vi "State Logic.vi"(0 "TLB' data in":refnum<class "{TMPL} TLB`.lvclass">, 1 "process state logic enable":bool, 5 "trigger queue in":refnum<queue>, 7 "action queue in":refnum<queue>, 11 "error in":errorcluster) -> (4 "TLB' data out":refnum<class "{TMPL} TLB`.lvclass">, 15 "error out":errorcluster)   [LabVIEW 2023, in "TLB` InstStu GPlugin Template.lvlib" / "{TMPL} TLB`.lvclass"]
doc: "Control process for TLB' template.\n\n<B>Input Parameters</B>\n\n<B>TLB' data in</B> is the templates' private data.\n\n<B>process state logic enable</B> enable state logic change.\n\n<B>trigger queue in</B> is a reference to a queue. Use the Create Trigger Queue function to obtain a queue reference. \n\n<B>action queue in</B> is a reference to a queue. Use the Create Action Queue function to obtain a queue reference. \n\n<B>timeout (ms)</B> queue timeout.\n\n<B>error in</B> describes error conditions that occur before this node runs. This input provides standard error in functionality.\n\n<B>Output Parameters</B>\n\n<B>TLB' data out</B> is the templates' private data.\n\n<B>error out</B> contains error information. This output provides standard error out functionality."
uses:
  {TMPL} TLB`.lvclass
  Application Components/Trigger API/System Trigger Element.ctl
  Application Components/Trigger API/System Trigger.ctl
  Core Components/Actions/System Action Element.ctl
  {TMPL} TLB`.lvclass/{TMPL} TLB`.ctl
  State.ctl
  Core Components/Error Handler/TLB` Error Handler.lvclass/TLB` Error Handler.ctl
  Core Components/Error Handler/accessors/Get Action Causing Error.vi
  Core Components/Error Handler/accessors/Get Originating State.vi
  Core Components/Error Handler/accessors/Get Destination State.vi
  Core Components/Error Handler/accessors/Get Executed System Actions.vi
  Core Components/Error Handler/accessors/Get Remaing System Actions.vi
  Core Components/Error Handler/Core/actions/support/Error FLUSH-LOG-DIALOG.vi
  Core Components/Error Handler/Core/actions/support/Error FLUSH-DIALOG.vi
  Application Components/Trigger API/{TMPL} Trigger API.lvlib
  Core Components/Error Handler/TLB` Error Handler.lvclass
  Core Components/Actions/Actions.lvlib
  TLB` InstStu GPlugin Template.lvlib
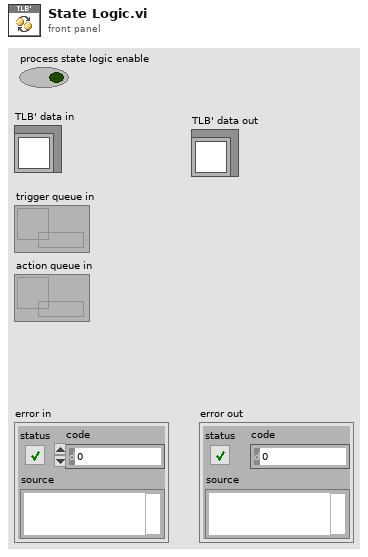
[diagram p1: front panel]
types:
  T1 = typedef "TLB` InstStu GPlugin Template.lvlib/{TMPL} TLB`.lvclass/State.ctl" = enum16{"<Startup>", "Idle", "Connected", "Monitoring", "<Shutdown>", "<Error>"}
  T2 = typedef "TLB` InstStu GPlugin Template.lvlib/{TMPL} Trigger API.lvlib/System Trigger.ctl" = enum16{"<None>", "Connect", "Start Acquisition", "Stop Acquisition", "Disconnect", "Load Configuration", "Save Configuration", "<Return to Safe State Actions>", "<Cache User Parameters>", "<Close Application>", "<Error>"}
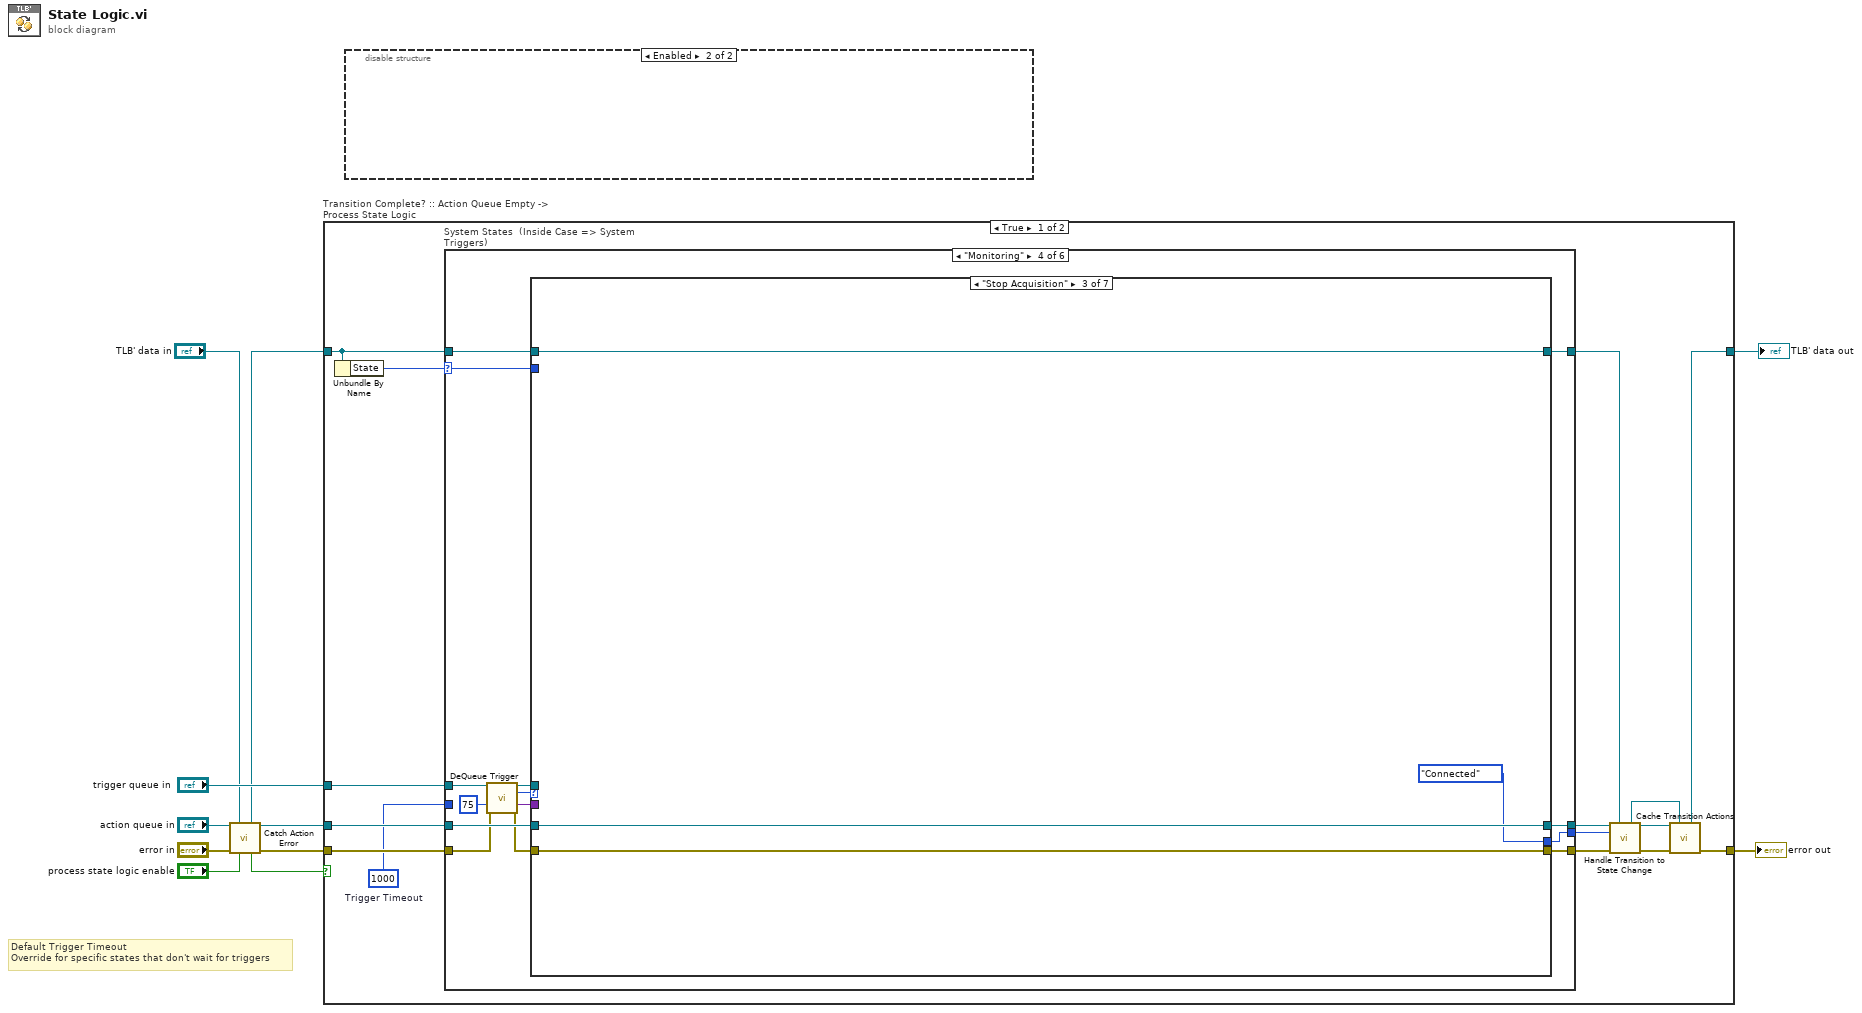
[diagram p0: block diagram]
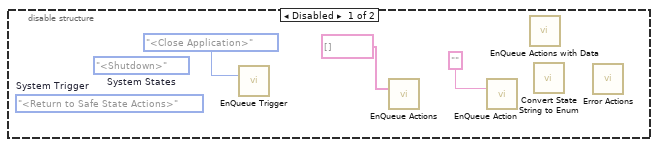
[diagram p2: hidden frame]
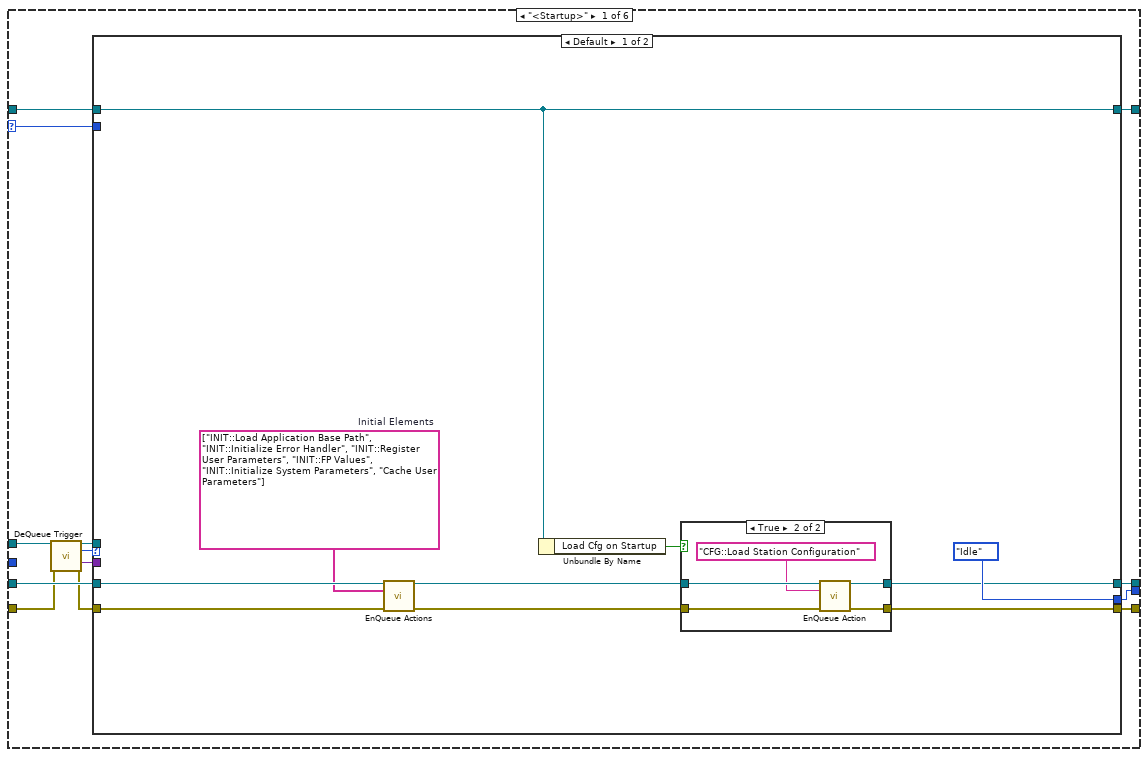
[diagram p3: hidden frame]
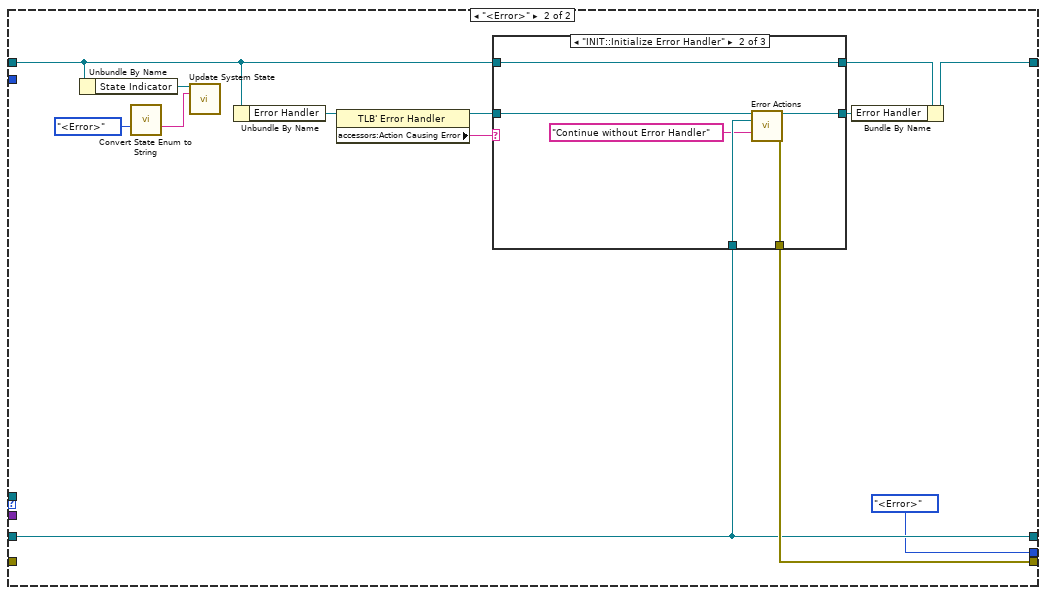
[diagram p5: hidden frame]
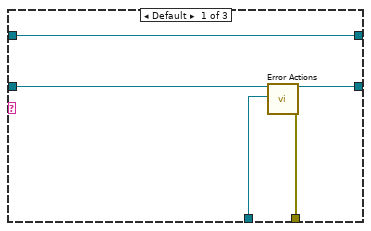
[diagram p6: hidden frame]
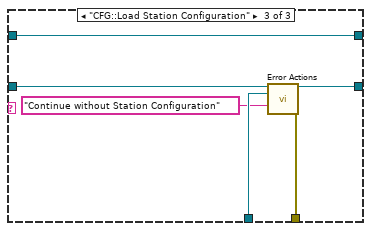
[diagram p7: hidden frame]
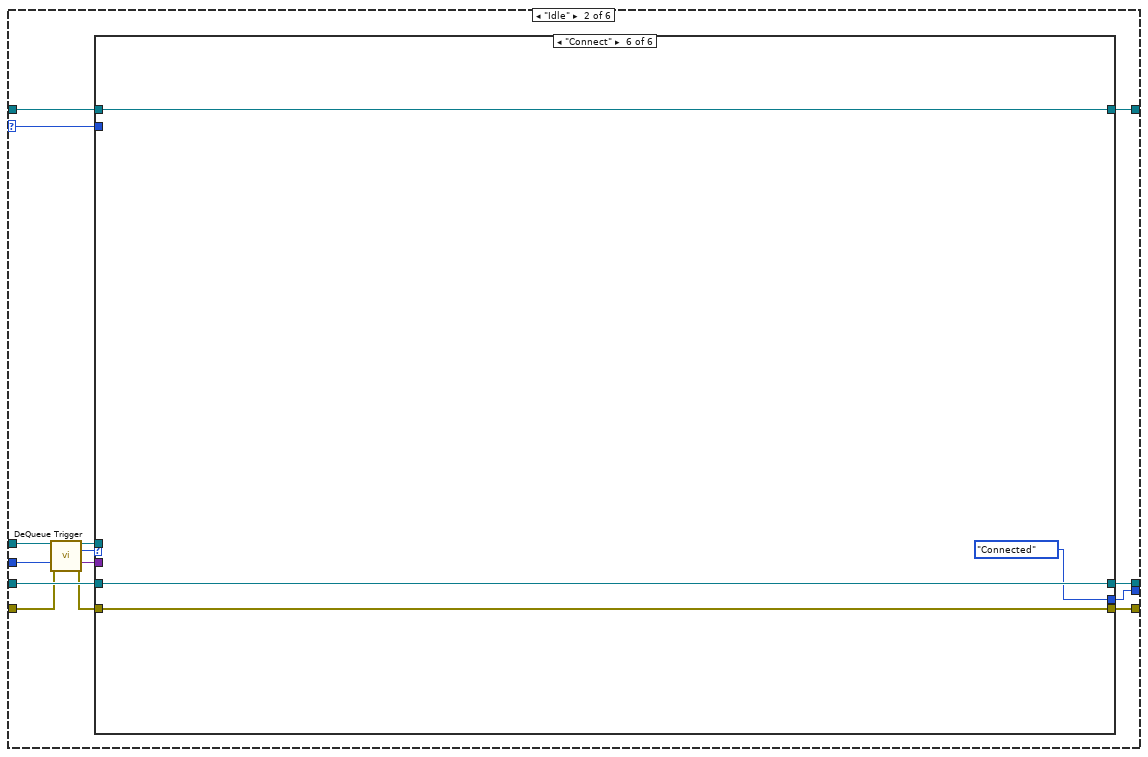
[diagram p8: hidden frame]
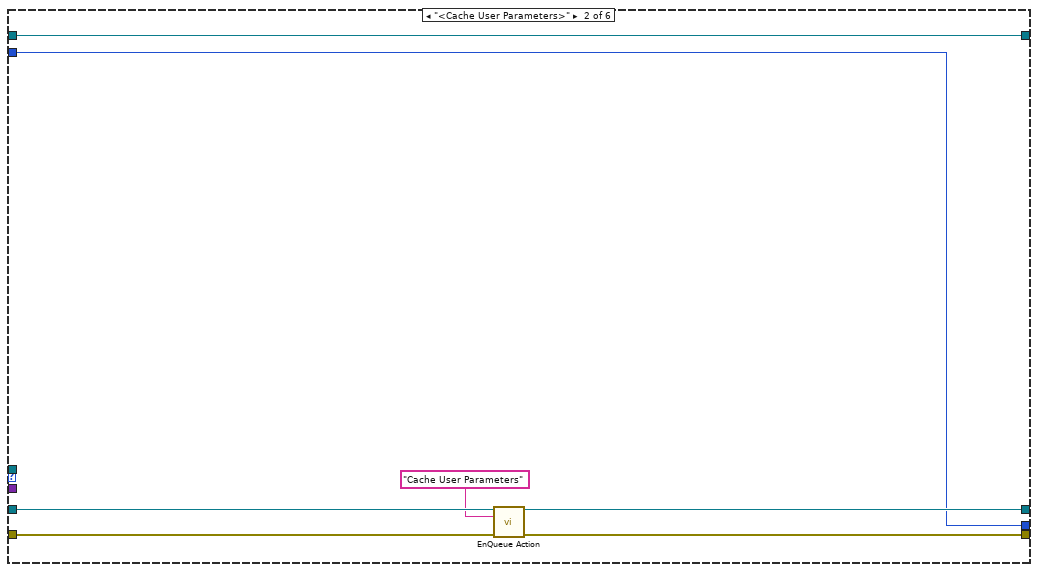
[diagram p10: hidden frame]
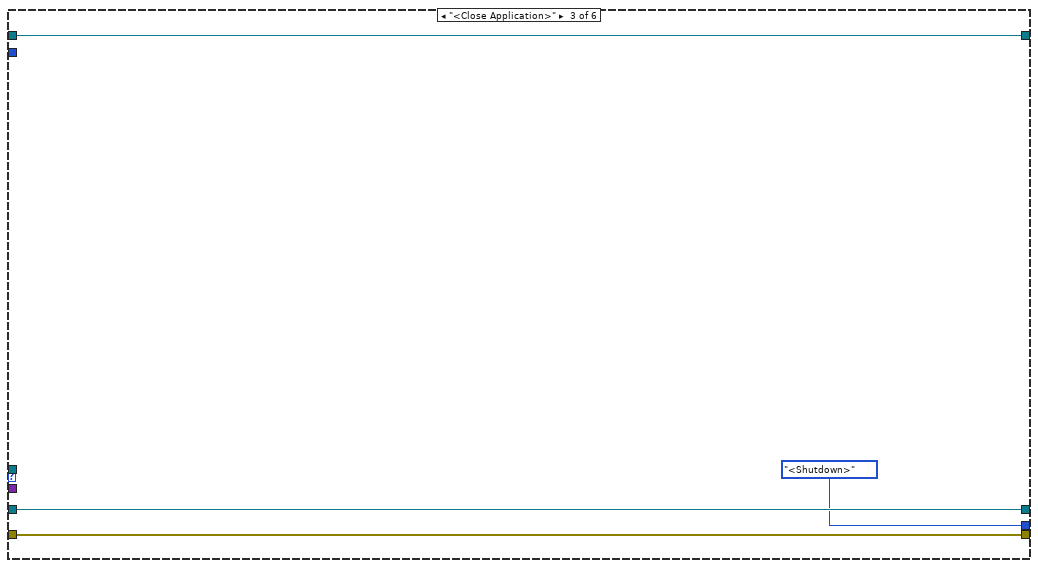
[diagram p11: hidden frame]
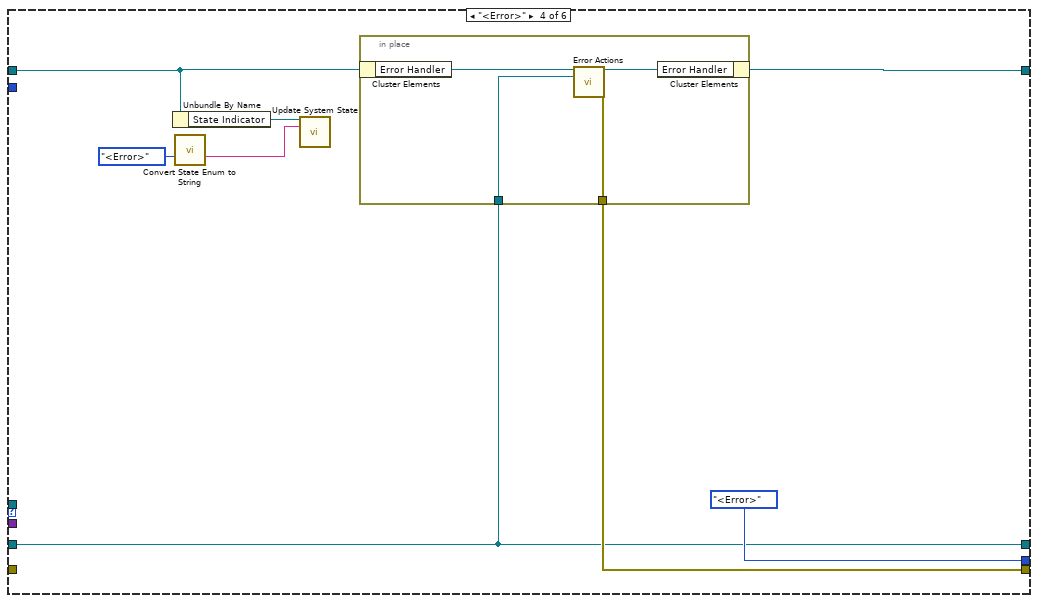
[diagram p12: hidden frame]
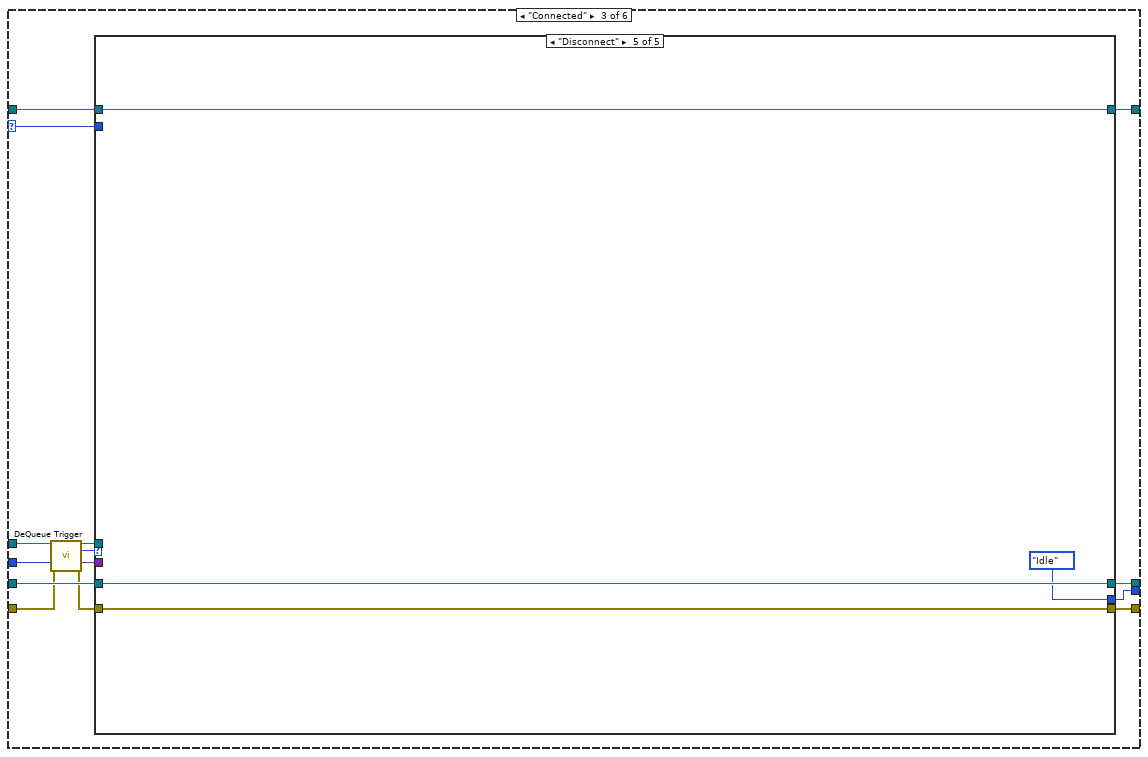
[diagram p14: hidden frame]
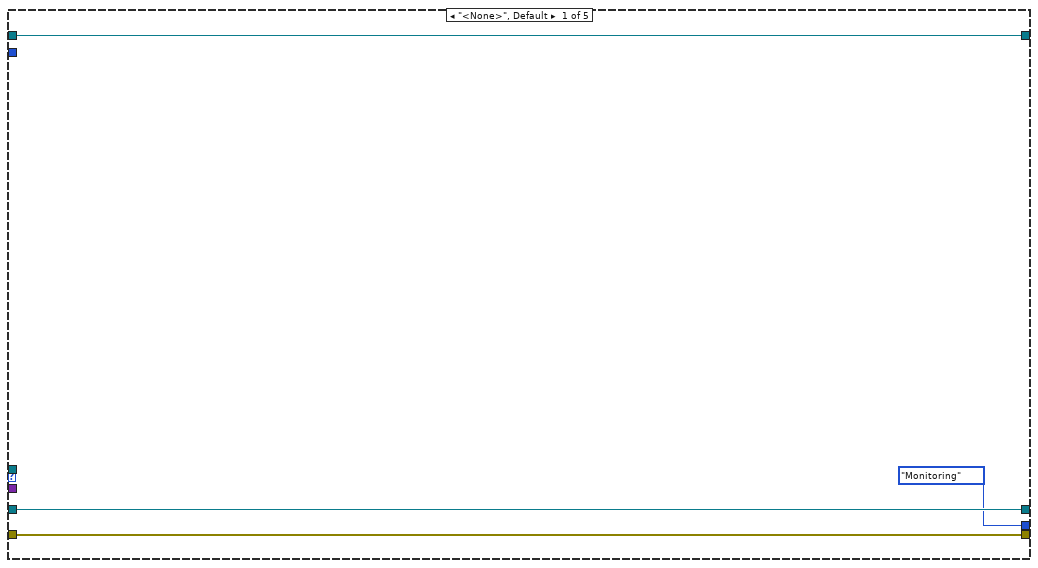
[diagram p15: hidden frame]
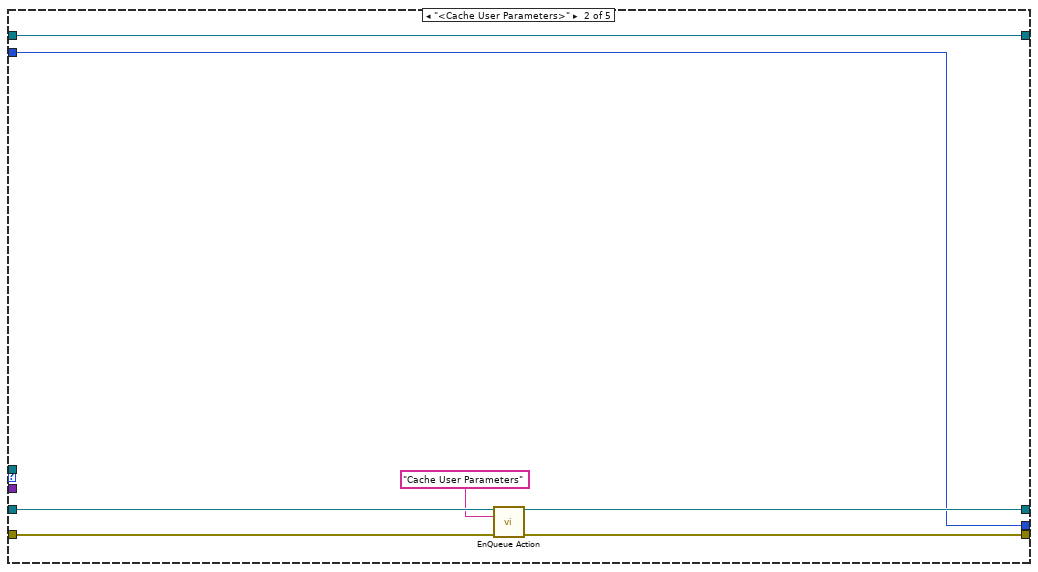
[diagram p16: hidden frame]
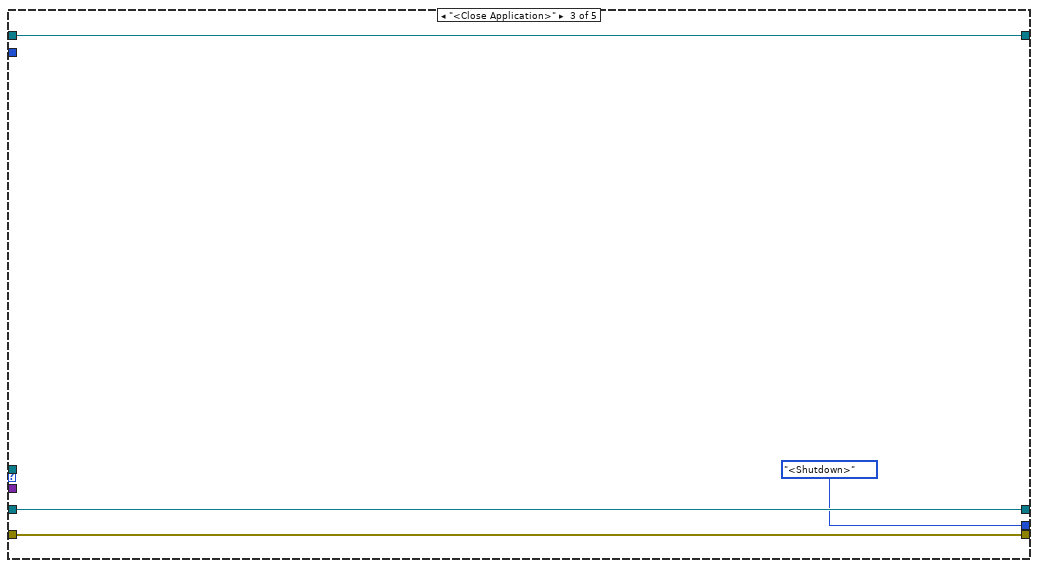
[diagram p17: hidden frame]
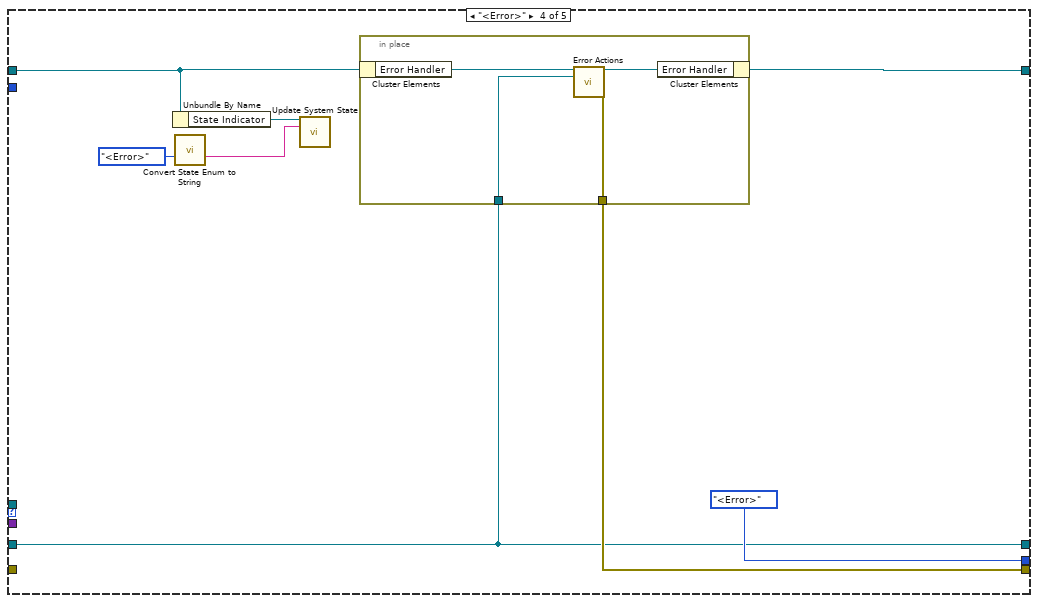
[diagram p18: hidden frame]
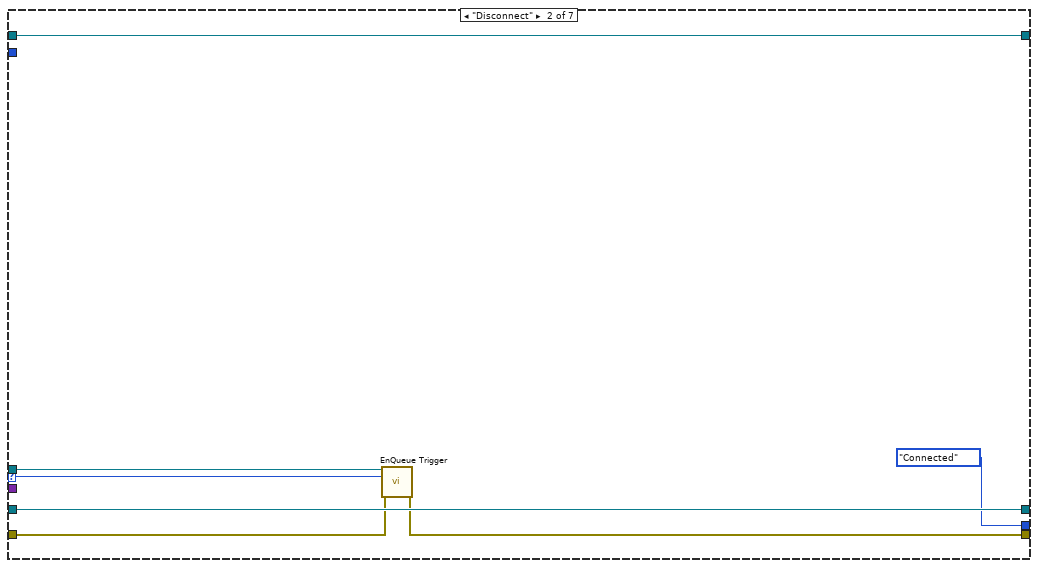
[diagram p20: hidden frame]
diagram:
  # "Default Trigger Timeout\nOverride for specific states that don't wait for triggers"
  n1 = call "Catch Action Error.vi"("action queue in"="action queue in", "TLB' Template in"="TLB' data in", "error in (no error)"="error in", "process state logic enable in"="process state logic enable") -> ("TLB' Template out"=w6:refnum<class "{TMPL} TLB`.lvclass">, "action queue in"=w2:refnum<queue>, "process state logic enable out"=w4:bool, "error out"=w7:errorcluster)  [unwired: 8 in]
  n2 = case "Transition Complete? :: Action Queue Empty -> Process State Logic" shown="True" w4 {
    tunnel: [w17 w343] -> w10
    tunnel: w6 -> [w22 w343]
    tunnel: w7 -> [w26 w344]
    tunnel: w2 -> [w25 _]
    tunnel: [w20 w344] -> w11
    tunnel: "trigger queue in" -> [w24 _]
    frame True {
      w18 = 1000  # Trigger Timeout
      n3 = Unbundle By Name(w22) -> ("State"=w19:T1)
      n4 = case "System States  (Inside Case => System Triggers)" shown="\"Monitoring\"" w19 {
        selector: w19 -> [w27 w89 w138 w183 w244 _]
        tunnel: [w33 w94 w143 w188 w242 w341] -> w15
        tunnel: w22 -> [w34 w95 w144 w189 w243 w341]
        tunnel: w26 -> [w32 w93 w142 w187 w241 w340]
        tunnel: w25 -> [w38 w99 w148 w193 w245 w339]
        tunnel: [w37 w98 w147 w192 w248 w337] -> w23
        tunnel: w24 -> [w39 w100 w149 w194 w249 _]
        tunnel: [w36 w97 w146 w191 w247 w338] -> w16
        tunnel: [w35 w96 w145 w190 w246 State."<Shutdown>" ("State")] -> w12
        tunnel: w18 -> [_ w88 w137 _ _ _]
        frame "<Startup>" {
          n5 = call "DeQueue Trigger.vi"("trigger queue in"=w39, "error in"=w32) -> ("trigger queue out"=w28:refnum<queue>, "system trigger"=w30:T2, "trigger data"=w29:variant, "error out"=w31:errorcluster)  [unwired: 10 in]
          n6 = case shown="Default" w30 {
            tunnel: w31 -> [w46 _]
            tunnel: w38 -> [w48 w67]
            tunnel: [w43 w68] -> w37
            tunnel: [w41 w67] -> w36
            tunnel: w29 -> [_ _]
            tunnel: [State."Idle" ("State") State."<Error>" ("State")] -> w35
            tunnel: w34 -> [w44 w58]
            tunnel: [w44 w69] -> w33
            tunnel: w28 -> [_ _]
            tunnel: w27 -> [_ _]
            frame Default {
              w47 = string[] ["INIT::Load Application Base Path", "INIT::Initialize Error Handler", "INIT::Register User Parameters", "INIT::FP Values", "INIT::Initialize System Parameters", "Cache User Parameters"]  # Initial Elements
              n7 = call "EnQueue Actions.vi"("action queue in"=w48, "actions"=w47, "error in"=w46) -> ("action queue out"=w42:refnum<queue>, "error out"=w45:errorcluster)  [unwired: 11 in]
              n8 = Unbundle By Name(w44) -> ("Load Cfg on Startup"=w40:bool)
              n9 = case shown="True" w40 {
                tunnel: w45 -> [w50 w56]
                tunnel: [w50 w55] -> w43
                tunnel: w42 -> [w51 w54]
                tunnel: [w51 w53] -> w41
                frame False {
                }
                frame True {
                  n10 = call "EnQueue Action.vi"("action queue in"=w54, "action"="CFG::Load Station Configuration", "error in"=w56) -> ("action queue out"=w53:refnum<queue>, "error out"=w55:errorcluster)  [unwired: 11 in]
                }
              }
            }
            frame "<Error>" {
              n11 = Unbundle By Name(w58) -> ("State Indicator"=w62:refnum<user-event>)
              n12 = call "Convert State Enum to String.vi"("state in"=State."<Error>") -> ("state out"=w61:string)  [unwired: 13 in, 1 out]
              n13 = call "Update System State.vi"("State Indicator"=w62, "system state message"=w61) -> ()  [unwired: 13 in, 1 out]
              n14 = Unbundle By Name(w58) -> ("Error Handler"=w64:refnum<class "TLB` Error Handler.lvclass">)
              n15 = property class="TLB' Error Handler"(reference=w64) -> (reference out=w63:refnum<class "TLB` Error Handler.lvclass">, "accessors:Action Causing Error"=w60:string)  [unwired: 1 in, 1 out]
              n16 = case shown="\"INIT::Initialize Error Handler\"" w60 {
                tunnel: [w72 w80 w86] -> w68
                tunnel: w67 -> [w71 w79 w85]
                tunnel: [w73 w78 w84] -> w65
                tunnel: w63 -> [w74 w77 w83]
                tunnel: w58 -> [w70 w75 w81]
                tunnel: [w70 w75 w81] -> w57
                frame Default {
                  n17 = call-poly "Error Actions.vi"("Error Handler in"=w74, "action queue in"=w71) -> ("Error Handler out"=w73:refnum<class "TLB` Error Handler.lvclass">, "error out"=w72:errorcluster)  [unwired: 12 in]
                }
                frame "INIT::Initialize Error Handler" {
                  n18 = call-poly "Error Actions.vi"("Error Handler in"=w77, "action queue in"=w79, "error button text (Return to Safe State)"="Continue without Error Handler") -> ("Error Handler out"=w78:refnum<class "TLB` Error Handler.lvclass">, "error out"=w80:errorcluster)  [unwired: 11 in]
                }
                frame "CFG::Load Station Configuration" {
                  n19 = call-poly "Error Actions.vi"("Error Handler in"=w83, "action queue in"=w85, "error button text (Return to Safe State)"="Continue without Station Configuration") -> ("Error Handler out"=w84:refnum<class "TLB` Error Handler.lvclass">, "error out"=w86:errorcluster)  [unwired: 11 in]
                }
              }
              n20 = Bundle By Name(cluster=w57, "Error Handler"=w65) -> (w69:refnum<class "{TMPL} TLB`.lvclass">)
            }
          }
        }
        frame "Idle" {
          n21 = call "DeQueue Trigger.vi"("trigger queue in"=w100, "timeout, ms (0)"=w88, "error in"=w93) -> ("trigger queue out"=w87:refnum<queue>, "system trigger"=w91:T2, "trigger data"=w90:variant, "error out"=w92:errorcluster)  [unwired: 9 in]
          n22 = case shown="\"Connect\"" w91 {
            tunnel: w92 -> [w103 w111 w114 _ w130 w135]
            tunnel: w99 -> [w104 w108 w115 w119 w131 w134]
            tunnel: [w103 w109 w114 w121 w130 w135] -> w98
            tunnel: [w104 w107 w115 w119 w131 w134] -> w97
            tunnel: w90 -> [_ _ _ _ _ _]
            tunnel: w95 -> [w102 w110 w113 w118 w129 w133]
            tunnel: [w101 w105 State."<Shutdown>" ("State") State."<Error>" ("State") w128 State."Connected" ("State")] -> w96
            tunnel: [w102 w110 w113 w120 w129 w133] -> w94
            tunnel: w89 -> [w101 w105 _ _ w128 _]
            tunnel: w87 -> [_ _ _ _ _ _]
            frame "<None>" {
            }
            frame "<Cache User Parameters>" {
              n23 = call "EnQueue Action.vi"("action queue in"=w108, "action"="Cache User Parameters", "error in"=w111) -> ("action queue out"=w107:refnum<queue>, "error out"=w109:errorcluster)  [unwired: 11 in]
            }
            frame "<Close Application>" {
            }
            frame "<Error>" {
              n24 = Unbundle By Name(w118) -> ("State Indicator"=w122:refnum<user-event>)
              n25 = call "Convert State Enum to String.vi"("state in"=State."<Error>") -> ("state out"=w116:string)  [unwired: 13 in, 1 out]
              n26 = call "Update System State.vi"("State Indicator"=w122, "system state message"=w116) -> ()  [unwired: 13 in, 1 out]
              n27 = in-place {
                in-place-border: [w125] -> w121
                in-place-border: w119 -> [w124]
                n28 = in-place-cluster #1(w118) -> ("Error Handler"=w127:refnum<class "TLB` Error Handler.lvclass">)
                n29 = call-poly "Error Actions.vi"("Error Handler in"=w127, "action queue in"=w124) -> ("Error Handler out"=w126:refnum<class "TLB` Error Handler.lvclass">, "error out"=w125:errorcluster)  [unwired: 12 in]
                n30 = in-place-cluster #1("Error Handler"=w126) -> (w120:refnum<class "{TMPL} TLB`.lvclass">)
              }
            }
            frame Default {
            }
            frame "Connect" {
            }
          }
        }
        frame "Connected" {
          n31 = call "DeQueue Trigger.vi"("trigger queue in"=w149, "timeout, ms (0)"=w137, "error in"=w142) -> ("trigger queue out"=w136:refnum<queue>, "system trigger"=w140:T2, "trigger data"=w139:variant, "error out"=w141:errorcluster)  [unwired: 9 in]
          n32 = case shown="\"Disconnect\"" w140 {
            tunnel: w141 -> [w152 w160 w163 _ w180]
            tunnel: w148 -> [w153 w157 w164 w168 w179]
            tunnel: [w152 w158 w163 w170 w180] -> w147
            tunnel: [w153 w156 w164 w168 w179] -> w146
            tunnel: w139 -> [_ _ _ _ _]
            tunnel: w144 -> [w151 w159 w162 w167 w178]
            tunnel: [State."Monitoring" ("State") w154 State."<Shutdown>" ("State") State."<Error>" ("State") State."Idle" ("State")] -> w145
            tunnel: [w151 w159 w162 w169 w178] -> w143
            tunnel: w138 -> [_ w154 _ _ _]
            tunnel: w136 -> [_ _ _ _ _]
            frame "<None>", Default {
            }
            frame "<Cache User Parameters>" {
              n33 = call "EnQueue Action.vi"("action queue in"=w157, "action"="Cache User Parameters", "error in"=w160) -> ("action queue out"=w156:refnum<queue>, "error out"=w158:errorcluster)  [unwired: 11 in]
            }
            frame "<Close Application>" {
            }
            frame "<Error>" {
              n34 = Unbundle By Name(w167) -> ("State Indicator"=w171:refnum<user-event>)
              n35 = call "Convert State Enum to String.vi"("state in"=State."<Error>") -> ("state out"=w165:string)  [unwired: 13 in, 1 out]
              n36 = call "Update System State.vi"("State Indicator"=w171, "system state message"=w165) -> ()  [unwired: 13 in, 1 out]
              n37 = in-place {
                in-place-border: [w174] -> w170
                in-place-border: w168 -> [w173]
                n38 = in-place-cluster #2(w167) -> ("Error Handler"=w176:refnum<class "TLB` Error Handler.lvclass">)
                n39 = call-poly "Error Actions.vi"("Error Handler in"=w176, "action queue in"=w173) -> ("Error Handler out"=w175:refnum<class "TLB` Error Handler.lvclass">, "error out"=w174:errorcluster)  [unwired: 12 in]
                n40 = in-place-cluster #2("Error Handler"=w175) -> (w169:refnum<class "{TMPL} TLB`.lvclass">)
              }
            }
            frame "Disconnect" {
            }
          }
        }
        frame "Monitoring" {
          n41 = call "DeQueue Trigger.vi"("trigger queue in"=w194, "timeout, ms (0)"=75, "error in"=w187) -> ("trigger queue out"=w182:refnum<queue>, "system trigger"=w185:T2, "trigger data"=w184:variant, "error out"=w186:errorcluster)  [unwired: 9 in]
          n42 = case shown="\"Stop Acquisition\"" w185 {
            selector: w185 -> [_ w203 _ _ _ _ _]
            tunnel: w186 -> [w197 w200 w206 w216 w219 _ w235]
            tunnel: w193 -> [w198 w205 w209 w213 w220 w224 w236]
            tunnel: [w197 w201 w206 w214 w219 w226 w235] -> w192
            tunnel: [w198 w205 w209 w212 w220 w224 w236] -> w191
            tunnel: w184 -> [_ _ _ _ _ _ _]
            tunnel: w189 -> [w196 w204 w208 w215 w218 w223 w234]
            tunnel: [w195 State."Connected" ("State") State."Connected" ("State") w210 State."<Shutdown>" ("State") State."<Error>" ("State") w233] -> w190
            tunnel: [w196 w204 w208 w215 w218 w225 w234] -> w188
            tunnel: w183 -> [w195 _ _ w210 _ _ w233]
            tunnel: w182 -> [_ w199 _ _ _ _ _]
            frame "<None>" {
            }
            frame "Disconnect" {
              n43 = call "EnQueue Trigger.vi"("trigger queue in"=w199, "system trigger"=w203, "error in"=w200) -> ("error out"=w201:errorcluster)  [unwired: 11 in, 1 out]
            }
            frame "Stop Acquisition" {
            }
            frame "<Cache User Parameters>" {
              n44 = call "EnQueue Action.vi"("action queue in"=w213, "action"="Cache User Parameters", "error in"=w216) -> ("action queue out"=w212:refnum<queue>, "error out"=w214:errorcluster)  [unwired: 11 in]
            }
            frame "<Close Application>" {
            }
            frame "<Error>" {
              n45 = Unbundle By Name(w223) -> ("State Indicator"=w227:refnum<user-event>)
              n46 = call "Convert State Enum to String.vi"("state in"=State."<Error>") -> ("state out"=w221:string)  [unwired: 13 in, 1 out]
              n47 = call "Update System State.vi"("State Indicator"=w227, "system state message"=w221) -> ()  [unwired: 13 in, 1 out]
              n48 = in-place {
                in-place-border: [w230] -> w226
                in-place-border: w224 -> [w229]
                n49 = in-place-cluster #3(w223) -> ("Error Handler"=w232:refnum<class "TLB` Error Handler.lvclass">)
                n50 = call-poly "Error Actions.vi"("Error Handler in"=w232, "action queue in"=w229) -> ("Error Handler out"=w231:refnum<class "TLB` Error Handler.lvclass">, "error out"=w230:errorcluster)  [unwired: 12 in]
                n51 = in-place-cluster #3("Error Handler"=w231) -> (w225:refnum<class "{TMPL} TLB`.lvclass">)
              }
            }
            frame Default {
            }
          }
        }
        frame "<Error>" {
          n52 = call "DeQueue Trigger.vi"("trigger queue in"=w249, "error in"=w241) -> ("trigger queue out"=w240:refnum<queue>, "system trigger"=w239:T2, "trigger data"=w237:variant, "error out"=w238:errorcluster)  [unwired: 10 in]
          n53 = case shown="\"<Close Application>\"" w239 {
            tunnel: w243 -> [w251 w254 w317 w333]
            tunnel: [w252 w264 w326 w332] -> w248
            tunnel: w238 -> [w252 w266 w327 w332]
            tunnel: w245 -> [w253 w267 w328 w335]
            tunnel: [w253 w265 w323 w335] -> w247
            tunnel: [w250 w263 w325 State."<Shutdown>" ("State")] -> w246
            tunnel: w240 -> [_ _ _ _]
            tunnel: w244 -> [w250 _ _ _]
            tunnel: w237 -> [_ _ _ _]
            tunnel: [w251 w262 w317 w333] -> w242
            frame Default {
            }
            frame "<Return to Safe State Actions>" {
              n54 = Unbundle By Name(w254) -> ("Error Handler"=w261:refnum<class "TLB` Error Handler.lvclass">)
              n55 = property class="TLB' Error Handler"(reference=w261) -> ("accessors:Originating State"=w256:string, "accessors:Action Causing Error"=w260:string, "accessors:Destination State"=w259:string, "accessors:Executed System Actions"=w258:string[], "accessors:Remaing System Actions"=w255:string[])  [unwired: 1 in, 2 out]
              n56 = call "Convert State String to Enum.vi"("state in"=w256) -> ("state out"=w257:T1)  [unwired: 13 in, 1 out]
              n57 = case shown="\"<Startup>\"" w257 {
                selector: w257 -> [w268 w275 _]
                tunnel: w267 -> [w271 w281 w314]
                tunnel: w266 -> [w269 w282 w313]
                tunnel: [w269 w280 w313] -> w264
                tunnel: [w271 w279 w314] -> w265
                tunnel: [w268 w278 State."<Shutdown>" ("State")] -> w263
                tunnel: w254 -> [w270 w272 w316]
                tunnel: [w270 w273 w316] -> w262
                tunnel: w260 -> [_ w277 _]
                tunnel: w259 -> [_ w274 _]
                tunnel: w258 -> [_ _ _]
                tunnel: w255 -> [_ w276 _]
                frame Default {
                }
                frame "<Startup>" {
                  n58 = case shown="\"INIT::Initialize Error Handler\"" w277 {
                    tunnel: w282 -> [w285 w298 w311]
                    tunnel: w281 -> [w286 w299 w312]
                    tunnel: [w285 w297 w310] -> w280
                    tunnel: [w286 w296 w309] -> w279
                    tunnel: [State."<Shutdown>" ("State") State."Idle" ("state out") State."Idle" ("state out")] -> w278
                    tunnel: w276 -> [_ w295 w308]
                    tunnel: w275 -> [_ w287 w301]
                    tunnel: w274 -> [_ _ _]
                    tunnel: w272 -> [w283 w289 w302]
                    tunnel: [w283 w288 w300] -> w273
                    frame Default {
                    }
                    frame "INIT::Initialize Error Handler" {
                      n59 = Search 1D Array(1D array=w295, element="Change State") -> (index of element=w293:i32)  [unwired: 1 in]
                      n60 = Delete From Array(array=w295, length=1, index=w293) -> (array with subset deleted=w294:string[])  [unwired: 1 out]
                      n61 = call "EnQueue Actions.vi"("action queue in"=w299, "actions"=w294, "error in"=w298) -> ("action queue out"=w296:refnum<queue>, "error out"=w297:errorcluster)  [unwired: 11 in]
                      n62 = Bundle By Name(cluster=w289, "State"=w287) -> (w288:refnum<class "{TMPL} TLB`.lvclass">)
                    }
                    frame "CFG::Load Station Configuration" {
                      n63 = Search 1D Array(1D array=w308, element="Change State") -> (index of element=w306:i32)  [unwired: 1 in]
                      n64 = Delete From Array(array=w308, length=1, index=w306) -> (array with subset deleted=w307:string[])  [unwired: 1 out]
                      n65 = call "EnQueue Actions.vi"("action queue in"=w312, "actions"=w307, "error in"=w311) -> ("action queue out"=w309:refnum<queue>, "error out"=w310:errorcluster)  [unwired: 11 in]
                      n66 = Bundle By Name(cluster=w302, "State"=w301) -> (w300:refnum<class "{TMPL} TLB`.lvclass">)
                    }
                  }
                }
                frame "<Shutdown>" {
                }
              }
            }
            frame "<Close Application>" {
              n67 = Unbundle By Name(w317) -> ("Error Handler"=w324:refnum<class "TLB` Error Handler.lvclass">)
              n68 = property class="TLB' Error Handler"(reference=w324) -> ("accessors:Originating State"=w322:string, "accessors:Action Causing Error"=w318:string, "accessors:Destination State"=w319:string, "accessors:Executed System Actions"=w320:string[])  [unwired: 1 in, 2 out]
              n69 = call "Convert State String to Enum.vi"("state in"=w322) -> ("state out"=w321:T1)  [unwired: 13 in, 1 out]
              n70 = case shown="Default" w321 {
                tunnel: w328 -> [w330]
                tunnel: w327 -> [w329]
                tunnel: [w329] -> w326
                tunnel: [w330] -> w323
                tunnel: [State."<Shutdown>" ("State")] -> w325
                tunnel: w318 -> [_]
                tunnel: w319 -> [_]
                tunnel: w320 -> [_]
                frame Default {
                }
              }
            }
            frame "<Error>" {
              # "If error errors' that is probably really bad and we should end the program"
            }
          }
        }
        frame "<Shutdown>" {
          n71 = call "EnQueue Actions.vi"("action queue in"=w339, "actions"=string[] ["Exit"], "error in"=w340) -> ("action queue out"=w338:refnum<queue>, "error out"=w337:errorcluster)  [unwired: 11 in]
        }
      }
      n72 = call "Handle Transition to State Change.vi"("action queue in"=w16, "TLB' Template in"=w15, "Destination State"=w12, "error in (no error)"=w23) -> ("TLB' Template out"=w14:refnum<class "{TMPL} TLB`.lvclass">, "action queue in"=w13:refnum<queue>, "error out"=w21:errorcluster)  [unwired: 9 in]
      n73 = call "Cache Transition Actions.vi"("action queue in"=w13, "TLB' Template in"=w14, "error in (no error)"=w21) -> ("TLB' Template out"=w17:refnum<class "{TMPL} TLB`.lvclass">, "error out"=w20:errorcluster)  [unwired: 11 in]
    }
    frame False {
    }
  }
  "error out" <- w11
  "TLB' data out" <- w10
  n74 = disable-structure shown="Enabled" {
    frame Disabled {
      (unwired) System_Trigger."<Return to Safe State Actions>"  # System Trigger
      (unwired) State."<Shutdown>"  # System States
      n75 = call "EnQueue Trigger.vi"("system trigger"=System_Trigger."<Close Application>" ("System Trigger")) -> ()  [unwired: 13 in, 2 out]
      n76 = call "EnQueue Actions.vi"("actions"=string[] [] ("message names")) -> ()  [unwired: 13 in, 2 out]
      n77 = call "EnQueue Action.vi"("action"="" ("Message Name")) -> ()  [unwired: 13 in, 2 out]
      n78 = call "EnQueue Actions with Data.vi"() -> ()  [unwired: 14 in, 2 out]
      n79 = call "Convert State String to Enum.vi"() -> ()  [unwired: 14 in, 2 out]
      n80 = call-poly "Error Actions.vi"() -> ()  [unwired: 14 in, 2 out]
    }
    frame Enabled {
    }
  }
